vi "EPS-Clear Error.vi"(8 "error in":errorcluster, 11 "EPS Setting In":T1) -> (0 "error out":errorcluster, 3 "EPS Setting Out":T1)   [LabVIEW 2018]
uses:
  Data Def/EPS-Setting.ctl
  Data Def/EPS-Access Mode.ctl
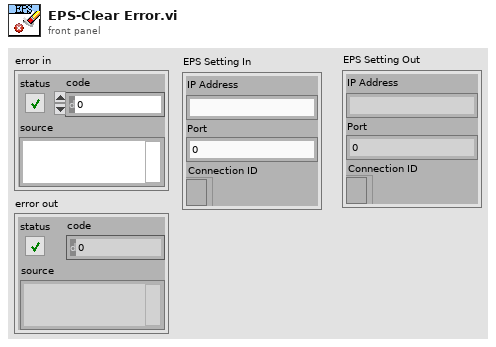
[diagram p1: front panel]
types:
  T1 = typedef "EPS-Setting.ctl" = cluster{"IP Address":string, "Port":u16, "Connection ID":refnum<k5>}
  T2 = typedef "EPS-Access Mode.ctl" = enum16{"Read", "Write"}
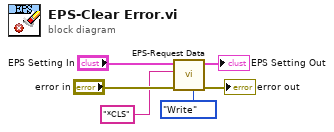
[diagram p0: block diagram]
diagram:
  n1 = call "EPS-Request Data.vi"("Access Mode"=EPS-Access_Mode."Write", "error in"="error in", "Requst Data"="*CLS", "EPS Setting In"="EPS Setting In") -> ("error out"=→"error out":errorcluster, "EPS Setting Out"=→"EPS Setting Out":T1)  [unwired: 5 in, 1 out]
